vi "_get mutiple control reference by name.vi"(4 "error in (no error)":errorcluster, 5 "Control names":string[](array[string]), 6 "Case sensitive (T)":bool, 7 "Control references":cluster{string, refnum<vi>}[](array[cluster])) -> (0 "error out":errorcluster, 2 "References":refnum<vi>[](array[refnum]))   [LabVIEW 2019]
doc: "This VI will give you a 1D array of control refrences by feeding it the output of the\" get reference to all controls\" VI and a 1D array of the names for the controls you would like a reference to."
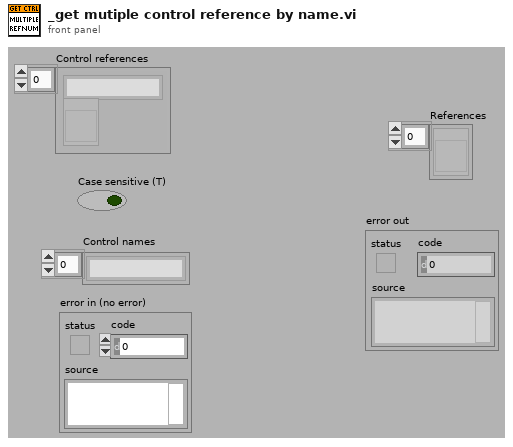
[diagram p1: front panel]
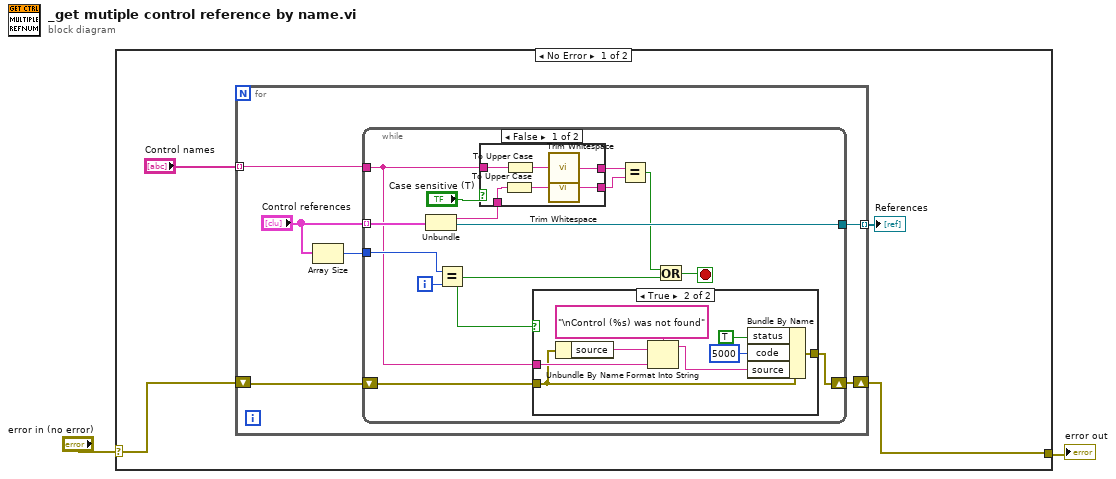
[diagram p0: block diagram]
diagram:
  n1 = case shown="No Error" "error in (no error)" {
    selector: "error in (no error)" -> [w4 w44]
    tunnel: [w3 w44] -> w2
    frame No Error {
      n2 = for {
        tunnel: [w10] -> w6 mode=indexing
        tunnel: "Control names" -> [w9] mode=indexing
        shift-right: [w7] -> w3
        shift-left: w4 -> [w8]
        n3 = Array Size(array="Control references") -> (size(s)=w12:i32)
        n4 = while {
          tunnel: "Control references" -> [w26] mode=indexing
          tunnel: [w25] -> w10
          tunnel: w9 -> [w15]
          tunnel: w12 -> [w23]
          shift-right: [w13] -> w7
          shift-left: w8 -> [w14]
          i -> [w24]
          stop <- w21 stop-if-true
          n5 = Unbundle(w26) -> (w18:string, w25:refnum<vi>)
          n6 = Equal?(x=w23, y=w24) -> (x = y?=w20:bool)
          n7 = case shown="False" "Case sensitive (T)" {
            tunnel: w15 -> [w32 w34]
            tunnel: w18 -> [w31 w33]
            tunnel: [w29 w34] -> w17
            tunnel: [w27 w33] -> w16
            frame False {
              n8 = To Upper Case(1:w31) -> (0:w28:string)
              n9 = To Upper Case(1:w32) -> (0:w30:string)
              n10 = call <vilib>:"Trim Whitespace.vi"("string"=w30) -> ("trimmed string"=w29:string)  [unwired: 1 in]
              n11 = call <vilib>:"Trim Whitespace.vi"("string"=w28) -> ("trimmed string"=w27:string)  [unwired: 1 in]
            }
            frame True {
            }
          }
          n12 = case shown="True" w20 {
            tunnel: w15 -> [_ w39]
            tunnel: w14 -> [w35 w37]
            tunnel: [w35 w38] -> w13
            frame False {
            }
            frame True {
              n13 = Unbundle By Name(w37) -> ("source"=w36:string)
              n14 = Format Into String(format string="\nControl (%s) was not found", initial string=w36, w39) -> (resulting string=w42:string)  [unwired: 1 in, 1 out]
              n15 = Bundle By Name(cluster=w37, "status"=TRUE, "code"=5000, "source"=w42) -> (w38:errorcluster)
            }
          }
          n16 = Equal?(x=w17, y=w16) -> (x = y?=w22:bool)
          n17 = Or(x=w22, y=w20) -> (x .or. y?=w21:bool)
        }
      }
      "References" <- w6
    }
    frame Error {
    }
  }
  "error out" <- w2
